vi "second_order_calculation.vi"() -> ()   [LabVIEW 2019]
panel:
  out "Numeric Output":dbl
  in  "Numeric 4":dbl
  in  "Numeric 3":dbl
  in  "Numeric 2":dbl
  in  "Numeric 1":dbl
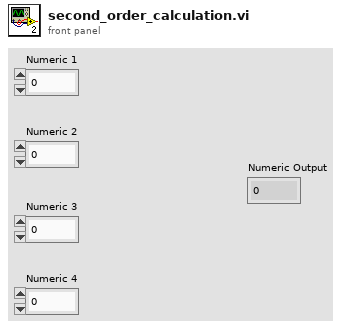
[diagram p1: front panel]
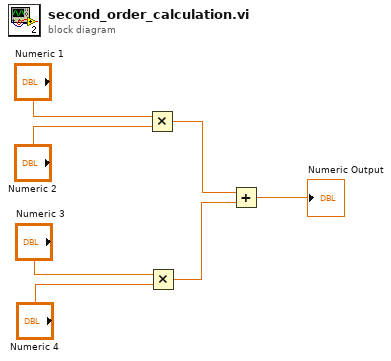
[diagram p0: block diagram]
diagram:
  n1 = Multiply(x="Numeric 1", y="Numeric 2") -> (x*y=w4:dbl)
  n2 = Multiply(x="Numeric 3", y="Numeric 4") -> (x*y=w3:dbl)
  n3 = Add(x=w4, y=w3) -> (x+y=→"Numeric Output":dbl)
